vi "LvMPDClient.vi"() -> ()   [LabVIEW 2012]
uses:
  <vilib>/Utility/sysdir.llb/System Directory Type.ctl
  <vilib>/Utility/miscctls.llb/LVPointTypeDef.ctl
  subvi/LvMPDC_Typdef_Setting.ctl
  subvi/LvMPDC_Global_Setting.vi
panel:
  out "Server":string="Title:" caption="Server:"
  out "flag playing":bool
  out "flag connect":bool
  out "flag setting":bool
  out "title":string="LvMPDClient"
  in  "Tree":string(tree)
  in  "List":i32(listbox)
  in  "volume":i32(slide) scale=0.0..100.0
  out "Total":string="59:59"
  out "Current":string="59:59"
  in  "Progress":dbl(slide) scale=0.0..272.0
  out "Artist":string="Artist:"
  out "Title":string="Title:" caption="Title:"
  in  "btn pause":bool
  in  "btn stop":bool
  in  "btn next":bool
  in  "btn prev":bool
  in  "btn play":bool
  # "MusicPlayerDaemon"
  # "http://www.musicpd.org/"
  # "file list"
  # "playlist"
  # "/"
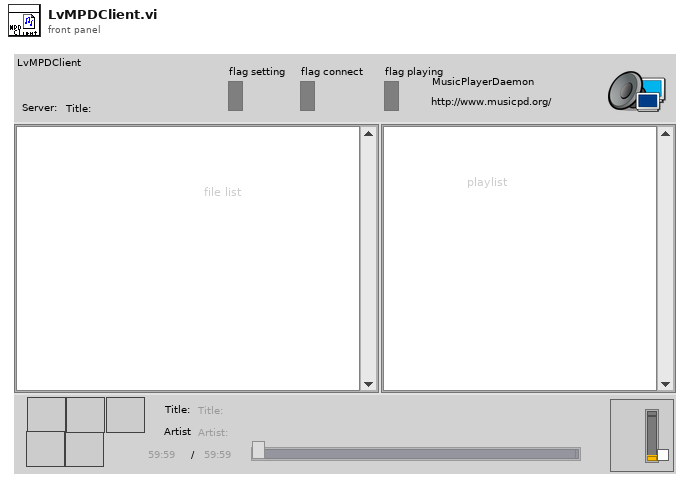
[diagram p1: front panel]
types:
  T1 = typedef "System Directory Type.ctl" = i32
  T2 = typedef "LVPointTypeDef.ctl" = cluster{"Horizontal":i16, "Vertical":i16}
  T3 = cluster{bool, "include Ctrl key?":bool, string}[]
  T4 = typedef "LvMPDC_Typdef_Setting.ctl" = cluster{"Server":string, "Port":u16}
  T5 = cluster{"配列[0]":i16, "配列[1]":i16, "配列[2]":i16, "配列[3]":i16}
  T6 = typedef "LvMPDC_Typdef_status.ctl" = cluster{"volume":i32, "repeat":i32, "random":i32, "single":i32, "consume":i32, "playlist":i32, "playlistlength":i32, "xfade":i32, "mixrampdb":dbl, "mixrampdelay":dbl, "state":enum16{"stop", "play", "pause"}, "song":i32, "songid":i32, "time":dbl, "elapsed":dbl, "bitrate":i32, "audio.samplerate":i32, "audio.bits":i32, "audio.channels":i32, "nextsong":i32, "nextsongid":i32}
  T7 = typedef "LvMPDC_Typdef_currentsong.ctl" = cluster{"file":path, "Last-Modified":string, "time":dbl, "Artist":string, "AlbumArtist":string, "Title":string, "Album":string, "Track":i32, "Date":string, "Genre":string, "Composer":string, "Pos":i32, "Id":i32}
  T8 = typedef "LVRectTypeDef.ctl" = cluster{"Left":i16, "Top":i16, "Right":i16, "Bottom":i16}
  T9 = enum32{"invalid app kind", "Development System", "Run Time System", "Student Edition", "Embedded LabVIEW", "Evaluation", "Custom"}
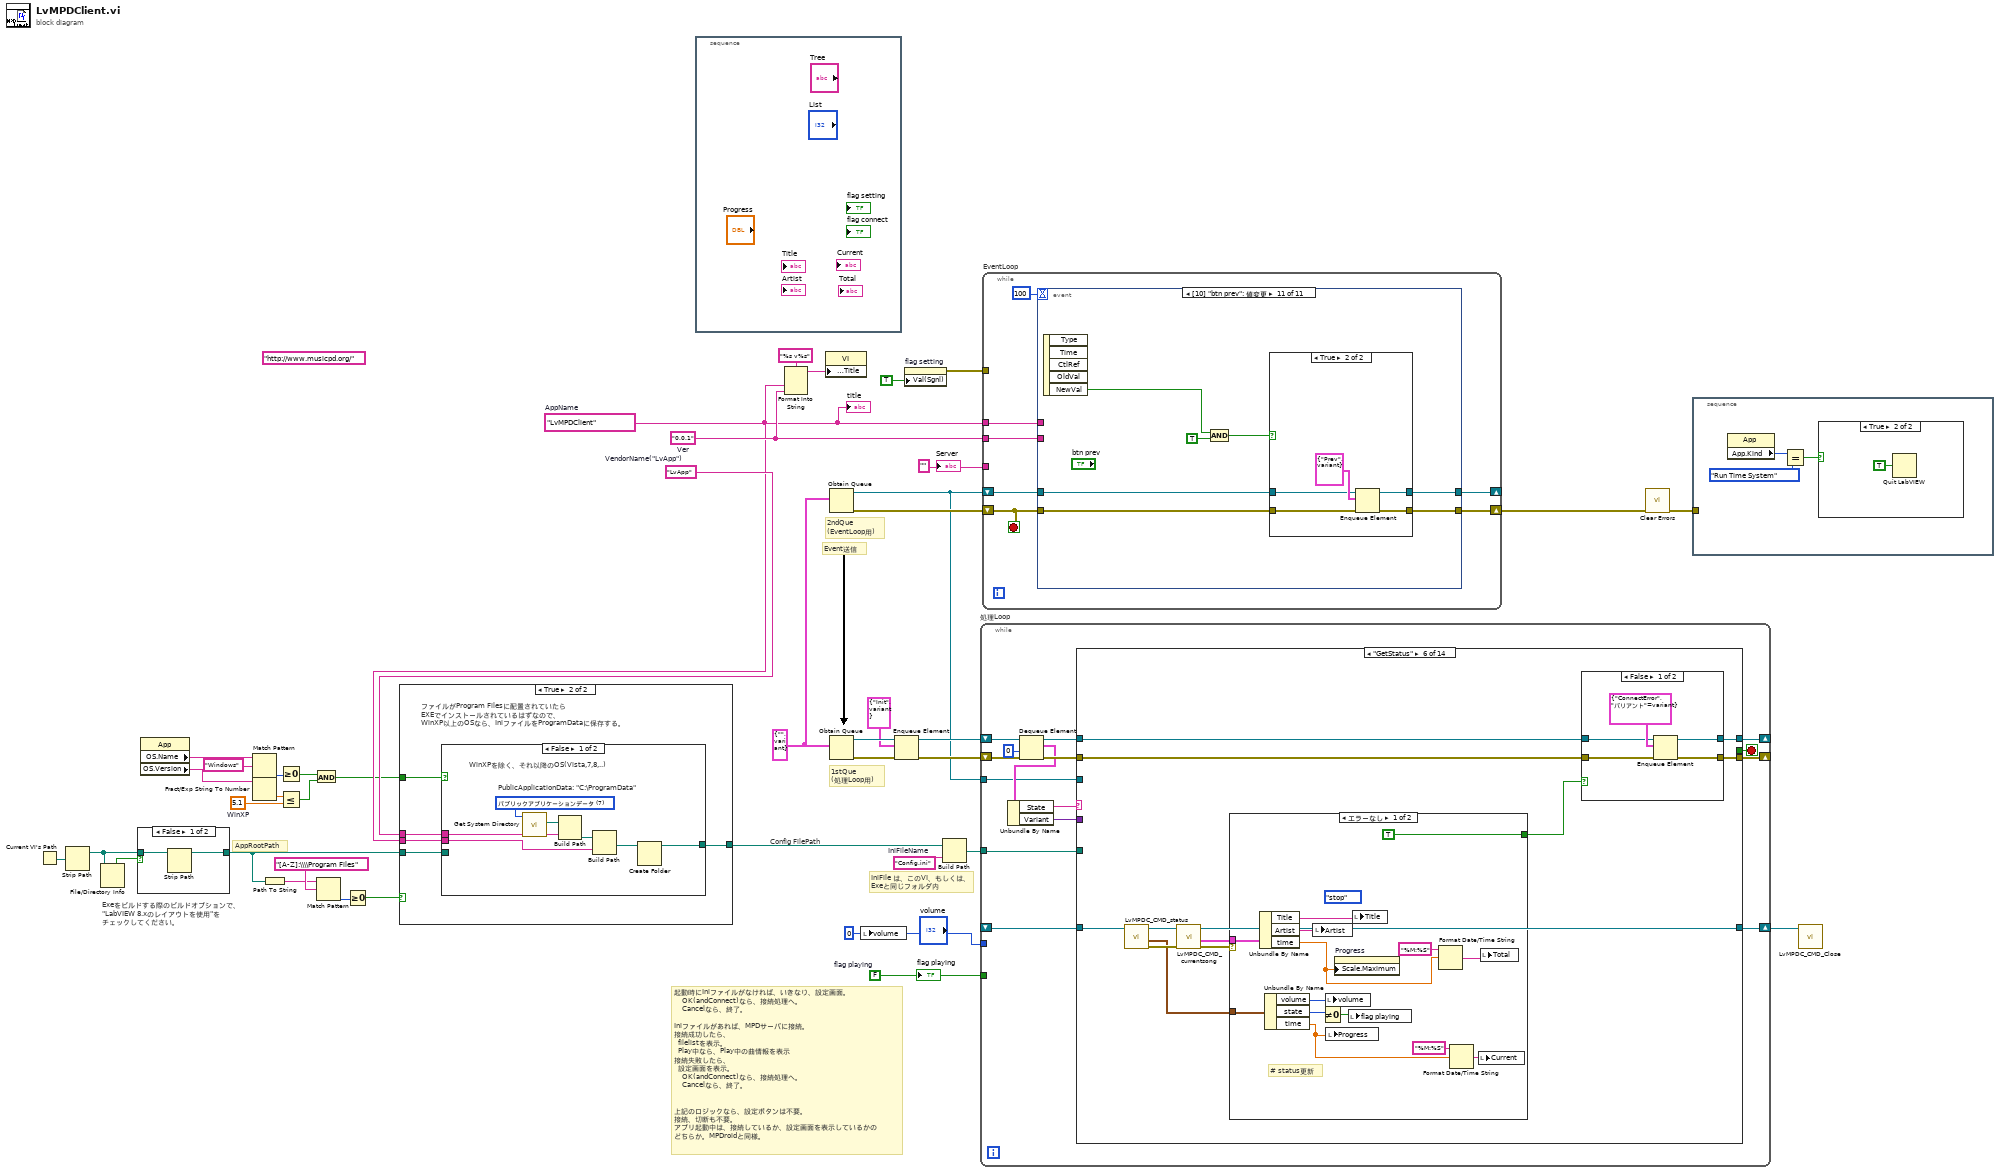
[diagram p0: block diagram]
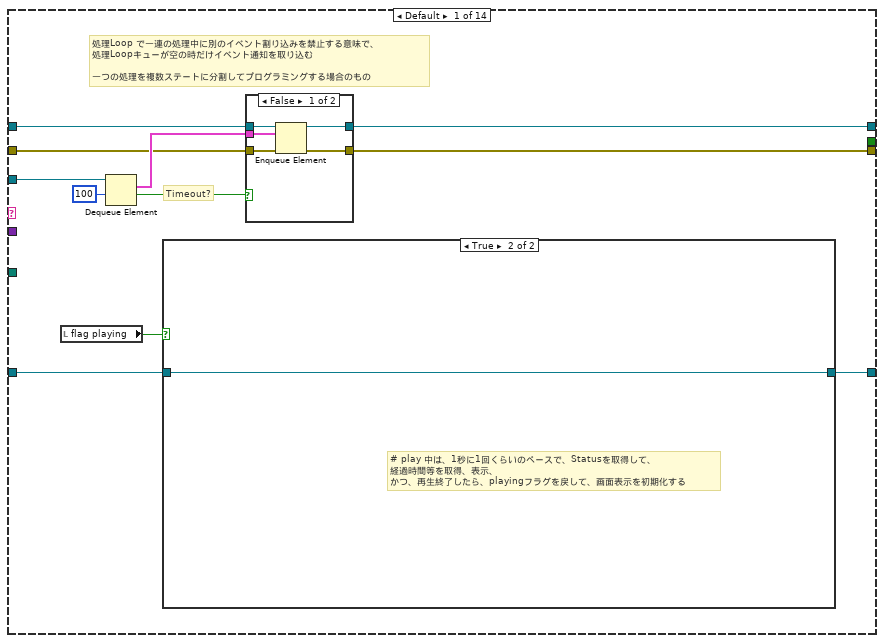
[diagram p6: hidden frame]
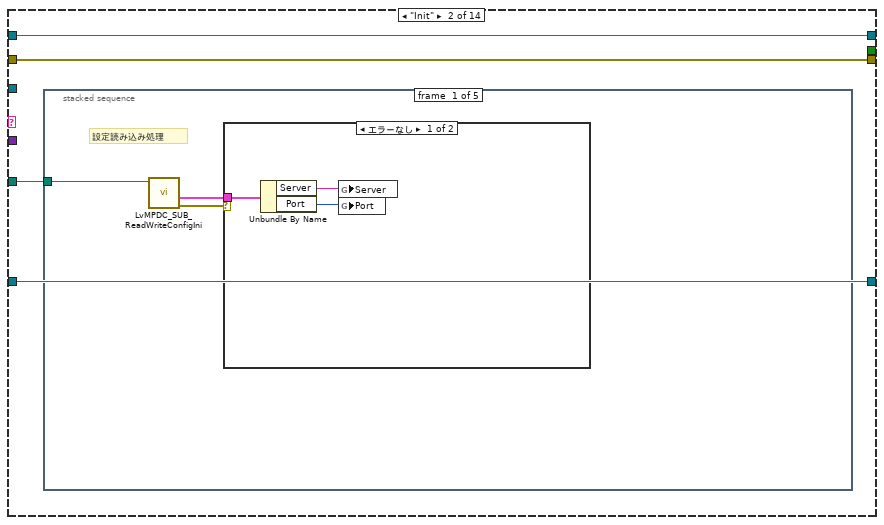
[diagram p9: hidden frame]
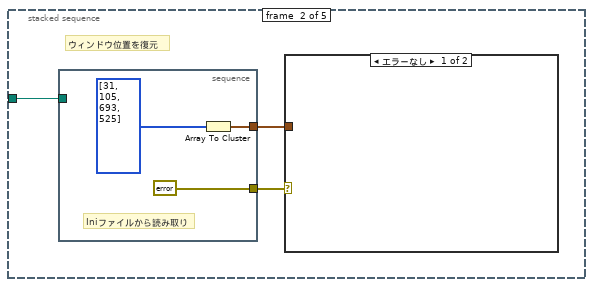
[diagram p11: hidden frame]
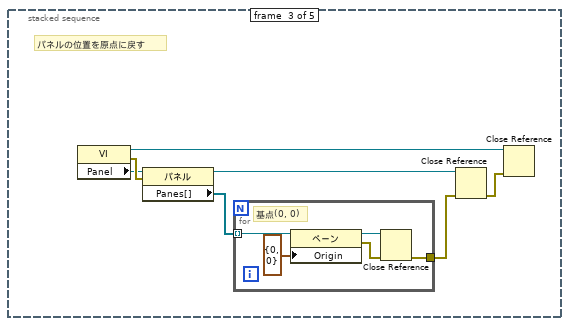
[diagram p13: hidden frame]
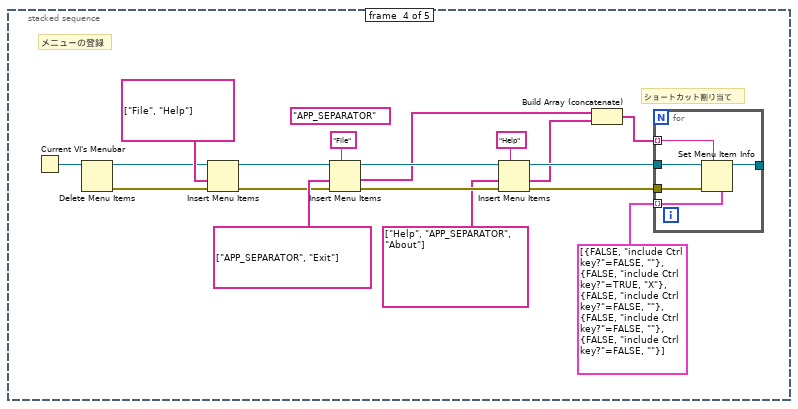
[diagram p14: hidden frame]
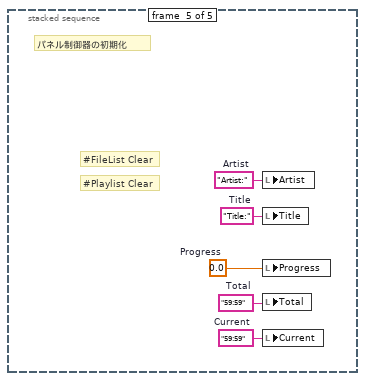
[diagram p15: hidden frame]
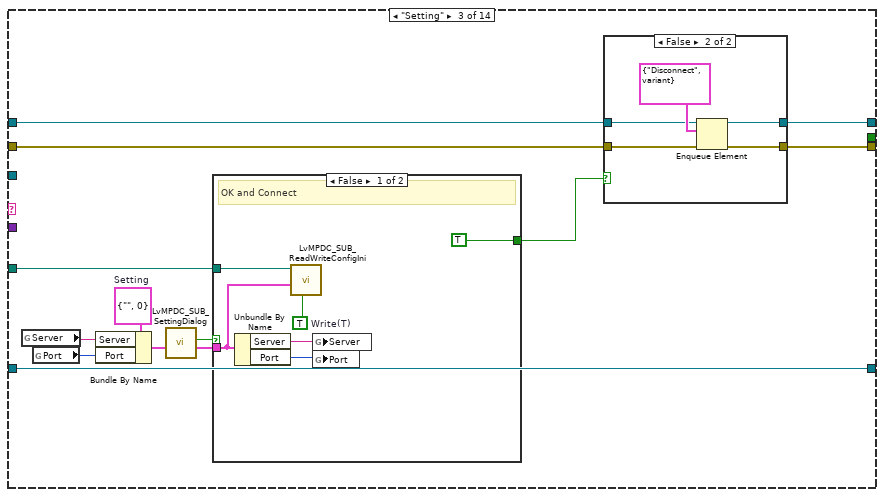
[diagram p16: hidden frame]
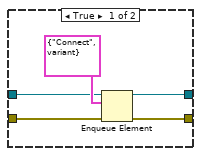
[diagram p17: hidden frame]
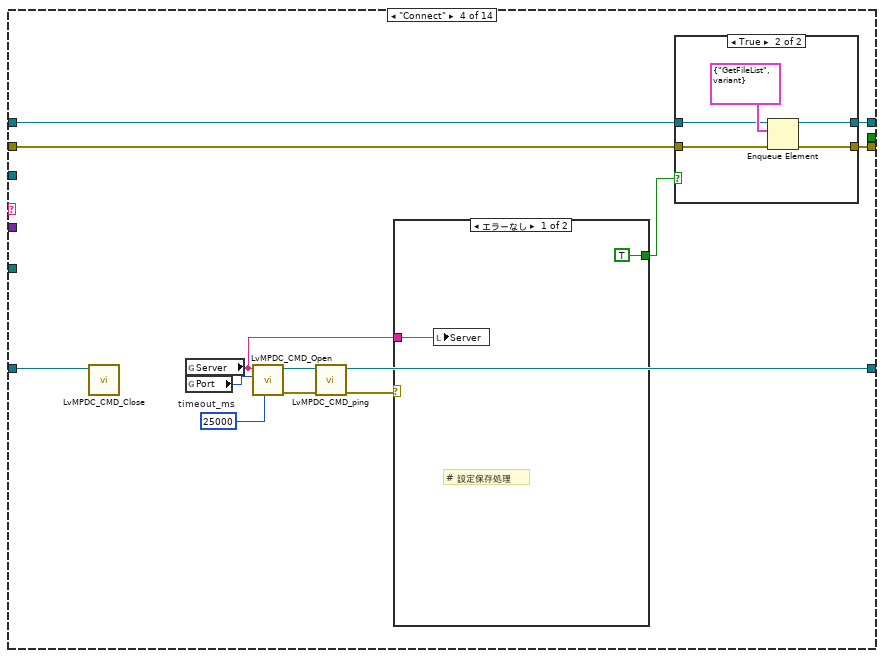
[diagram p19: hidden frame]
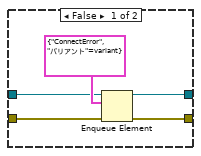
[diagram p20: hidden frame]
diagram:
  w1 = 0 ("volume")
  w2 = "" ("Server")
  w3 = FALSE  # flag playing
  (unwired) "http://www.musicpd.org/" ("aboud MPD")
  w17 = "LvApp"  # VendorName("LvApp")
  w22 = 5.1  # WinXP
  w27 = "Config.ini"  # IniFileName
  w30 = "0.0.1"  # Ver
  w16 = "LvMPDClient"  # AppName
  w41 = cluster{"State":string, "Variant":variant} {"State"="", "Variant"=variant}
  # "起動時にIniファイルがなければ、いきなり、設定画面。\n    OK(andConnect)なら、接続処理へ。\n    Cancelなら、終了。\n\nIniファイルがあれば、MPDサーバに接続。\n接続成功したら、\n  filelistを表示。\n  Play中なら、Play中の曲情報を表示\n接続失敗したら、\n  設定画面を表示。\n    OK(andConnect)なら、接続処理へ。\n    Cancelなら、終了。\n\n\n上記のロジックなら、設定ボタンは不要。\n接続、切断も不要。\nアプリ起動中は、接続しているか、設定画面を表示しているかの\nどちらか。MPDroidと同様。"
  # "Exeをビルドする際のビルドオプションで、\n\"LabVIEW 8.xのレイアウトを使用\"を\nチェックしてください。"
  # "Config FilePath"
  # "AppRootPath"
  # "IniFile は、このVI、もしくは、\nExeと同じフォルダ内"
  # "2ndQue\n(EventLoop用)"
  # "1stQue\n(処理Loop用)"
  # "Event送信"
  n1 = Current VI's Path() -> (path=w13:path)
  n2 = Strip Path(path=w13) -> (stripped path=w14:path)  [unwired: 1 out]
  n3 = File/Directory Info(path=w14) -> (directory=w15:bool)  [unwired: 1 in, 6 out]
  n4 = case shown="FALSE" w15 {
    tunnel: w14 -> [w43 w44]
    tunnel: [w42 w44] -> w10
    frame False {
      n5 = Strip Path(path=w43) -> (stripped path=w42:path)  [unwired: 1 out]
    }
    frame True {
    }
  }
  n6 = property class="App"() -> ("OS.Name"=w26:string, "OS.Version"=w24:string)  [unwired: 2 in, 2 out]
  n7 = Match Pattern(string=w26, regular expression="Windows" ("正規表現")) -> (offset past match=w21:i32)  [unwired: 1 in, 3 out]
  n8 = Fract/Exp String To Number(string=w24) -> (number=w23:dbl)  [unwired: 3 in, 1 out]
  n9 = Path To String(path=w10) -> (string=w9:string)
  n10 = Greater Or Equal To 0?(x=w21) -> (x >= 0?=w20:bool)
  n11 = Less Or Equal?(x=w23, y=w22) -> (x <= y?=w19:bool)
  n12 = And(x=w20, y=w19) -> (x .and. y?=w12:bool)
  n13 = Match Pattern(string=w9, regular expression="[A-Z]:\\\\Program Files" ("正規表現")) -> (offset past match=w8:i32)  [unwired: 1 in, 3 out]
  n14 = Greater Or Equal To 0?(x=w8) -> (x >= 0?=w7:bool)
  n15 = case shown="TRUE" w7 {
    tunnel: w16 -> [_ w50]
    tunnel: [w45 w48] -> w18
    tunnel: w17 -> [_ w49]
    tunnel: w12 -> [_ w47]
    tunnel: w10 -> [w45 w46]
    frame False {
      # "ファイルがProgram Filesに配置されていなかったら\n開発システムでソースから実行しているか、\nExeで適当なフォルダから実行されているので、\nIniファイルは、EXE, またはTop VI と同じ場所に保存"
    }
    frame True {
      # "ファイルがProgram Filesに配置されていたら\nEXEでインストールされているはずなので、\nWinXP以上のOSなら、IniファイルをProgramDataに保存する。"
      n16 = case shown="FALSE" w47 {
        tunnel: w50 -> [w54 _]
        tunnel: w49 -> [w52 _]
        tunnel: [w51 w58] -> w48
        tunnel: w46 -> [_ w58]
        frame False {
          w57 = T1 7 items=["ユーザホーム"=0, "ユーザデスクトップ"=1, "ユーザドキュメント"=2, "ユーザアプリケーションデータ"=3, "ユーザ設定"=4, "ユーザ一時"=5, "パブリックドキュメント"=6, "パブリックアプリケーションデータ"=7, "パブリック環境設定"=8, "パブリックキャッシュ"=13, "システムコアライブラリ"=9, "システムインストールされたライブラリ"=10, "アプリケーションファイル"=11, "ブート容量ルート"=12] ("system directory type")
          # "PublicApplicationData: \"C:\\ProgramData\""
          # "WinXPを除く、それ以降のOS(Vista,7,8,..)"
          n17 = call <vilib>:"Get System Directory.vi"("system directory type"=w57) -> ("system directory"=w56:path)  [unwired: 10 in]
          n18 = Build Path(base path=w56, name or relative path=w52) -> (appended path=w55:path)
          n19 = Build Path(base path=w55, name or relative path=w54) -> (appended path=w53:path)
          n20 = Create Folder(path (use dialog)=w53) -> (created path=w51:path)  [unwired: 2 in, 2 out]
        }
        frame True {
        }
      }
    }
  }
  n21 = stacked-sequence {
    frame #0 {
    }
  }
  n22 = Format Into String(format string="%s v%s" ("形式文字列"), w16, w30) -> (resulting string=w28:string)  [unwired: 2 in, 1 out]
  n23 = property class="VI"("Front Panel.Title"=w28) -> ()  [unwired: 2 in, 2 out]
  n24 = Obtain Queue(element data type=w41) -> (queue out=w34:refnum<queue>, error out=w40:errorcluster)  [unwired: 4 in, 1 out]
  n25 = Obtain Queue(element data type=w41) -> (queue out=w39:refnum<queue>, error out=w37:errorcluster)  [unwired: 4 in, 1 out]
  n26 = local write "volume"(w1) -> ()
  n27 = Enqueue Element(queue=w39, element=cluster{string, "バリアント":variant} {"Init", "バリアント"=variant}, error in (no error)=w37) -> (queue out=w38:refnum<queue>, error out=w36:errorcluster)  [unwired: 1 in, 1 out]
  n28 = property on="flag setting" class="Bool （指定）"("Val(Sgnl)"=TRUE) -> (error out=w5:errorcluster)  [unwired: 2 in, 1 out]
  n29 = Build Path(base path=w18, name or relative path=w27) -> (appended path=w31:path)
  n30 = while "処理Loop" {
    shift-right: [w68] -> _
    shift-left: w38 -> [w73]
    shift-right: [w67] -> _
    shift-left: w36 -> [w70]
    tunnel: w34 -> [w63]
    tunnel: w31 -> [w61]
    shift-right: [w60] -> w4
    shift-left: _ -> [w59]
    tunnel: w3 -> [_]
    tunnel: w1 -> [_]
    stop <- w62 stop-if-true
    n31 = Dequeue Element(queue=w73, timeout in ms (-1)=0 ("タイムアウト（ms）（-1）"), error in (no error)=w70) -> (queue out=w72:refnum<queue>, element=w66:cluster{"State":string, "Variant":variant}, error out=w69:errorcluster)  [unwired: 1 out]
    n32 = Unbundle By Name(w66) -> ("State"=w65:string, "Variant"=w64:variant)
    n33 = case shown="\"GetStatus\"" w65 {
      tunnel: w72 -> [w81 w97 w159 w186 w208 w233 w271 w297 w323 w348 w373 w396 w401 w411]
      tunnel: w63 -> [w84 _ _ _ _ _ _ _ _ _ _ _ _ w409]
      tunnel: w69 -> [w79 w96 w157 w185 w207 w232 w270 w296 w322 w347 w372 w395 w400 w408]
      tunnel: [w80 w97 w158 w184 w206 w231 w269 w295 w321 w346 w371 w393 w398 refnum<queue> refnum ("queue out")] -> w68
      tunnel: [w78 w96 w156 w183 w205 w230 w268 w294 w320 w345 w370 w394 w399 w407] -> w67
      tunnel: w64 -> [_ _ _ _ _ _ _ _ _ _ _ _ _ _]
      tunnel: [_ _ _ _ _ _ _ _ _ _ _ _ _ TRUE] -> w62
      tunnel: w61 -> [_ w95 w150 _ _ _ _ _ _ _ _ _ _ w406]
      tunnel: [w75 w94 w160 w189 w209 w225 w265 w291 w317 w342 w367 w392 w403 w405] -> w60
      tunnel: w59 -> [w76 w94 w160 w188 w209 w228 w266 w292 w318 w343 w368 w392 w404 w405]
      frame Default {
        # "Timeout?"
        # "処理Loop で一連の処理中に別のイベント割り込みを禁止する意味で、\n処理Loopキューが空の時だけイベント通知を取り込む\n\n一つの処理を複数ステートに分割してプログラミングする場合のもの"
        n34 = local read "flag playing"() -> (w74:bool)
        n35 = Dequeue Element(queue=w84, timeout in ms (-1)=100 ("タイムアウト（ms）（-1）")) -> (element=w82:cluster{"State":string, "Variant":variant}, timed out?=w77:bool)  [unwired: 1 in, 2 out]
        n36 = case shown="TRUE" w74 {
          tunnel: w76 -> [w85 w86]
          tunnel: [w85 w86] -> w75
          frame False {
          }
          frame True {
            # "# play 中は、1秒に1回くらいのペースで、Statusを取得して、\n経過時間等を取得、表示、\nかつ、再生終了したら、playingフラグを戻して、画面表示を初期化する"
          }
        }
        n37 = case shown="FALSE" w77 {
          tunnel: w82 -> [w91 _]
          tunnel: w81 -> [w90 w93]
          tunnel: [w89 w93] -> w80
          tunnel: w79 -> [w88 w92]
          tunnel: [w87 w92] -> w78
          frame False {
            n38 = Enqueue Element(queue=w90, element=w91, error in (no error)=w88) -> (queue out=w89:refnum<queue>, error out=w87:errorcluster)  [unwired: 1 in, 1 out]
          }
          frame True {
          }
        }
      }
      frame "Init" {
        n39 = stacked-sequence {
          tunnel: w95 -> [w100 w104 _ _ _]
          frame #0 {
            # "設定読み込み処理"
            n40 = call "LvMPDC_SUB_ReadWriteConfigIni.vi"("ConfigIni filepath"=w100) -> ("error out"=w99:errorcluster, "Config out"=w98:T4)  [unwired: 9 in]
            n41 = case shown="エラーなし" w99 {
              tunnel: w98 -> [w101 _]
              frame No Error {
                n42 = Unbundle By Name(w101) -> ("Server"=w103:string, "Port"=w102:u16)
                n43 = global write "LvMPDC_Global_Setting.vi" "Server"(w103) -> ()
                n44 = global write "LvMPDC_Global_Setting.vi" "Port"(w102) -> ()
              }
              frame Error {
              }
            }
          }
          frame #1 {
            # "ウィンドウ位置を復元"
            n45 = stacked-sequence {
              tunnel: [w107] -> w106
              tunnel: [errorcluster {"status"=FALSE, "code"=0, "source"=""} ("error in (no error)")] -> w105
              tunnel: w104 -> [_]
              frame #0 {
                # "Iniファイルから読み取り"
                n46 = Array To Cluster(array=i16[] [31, 105, 693, 525] ("配列")) -> (cluster=w107:T5)
              }
            }
            n47 = case shown="エラーなし" w105 {
              tunnel: w106 -> [_ _]
              frame No Error {
              }
              frame Error {
              }
            }
          }
          frame #2 {
            # "パネルの位置を原点に戻す"
            n48 = property class="VI"() -> (reference out=w113:refnum<vi>, error out=w116:errorcluster, "Panel"=w110:refnum<vi>)  [unwired: 2 in]
            n49 = property on="プロパティノード" class="パネル"(reference=w110, error in=w116) -> (reference out=w112:refnum<vi>, "Panes[]"=w111:refnum<vi>[])  [unwired: 1 out]
            n50 = for {
              tunnel: w111 -> [w121] mode=indexing
              tunnel: [w118] -> w114
              # "基点(0, 0)"
              n51 = property on="プロパティノード" class="ペーン"(reference=w121, "Origin"=T2 {"Horizontal"=0, "Vertical"=0} ("原点")) -> (reference out=w120:refnum<vi>, error out=w119:errorcluster)  [unwired: 1 in]
              n52 = Close Reference(reference=w120, error in (no error)=w119) -> (error out=w118:errorcluster)
            }
            n53 = Close Reference(reference=w112, error in (no error)=w114) -> (error out=w115:errorcluster)
            n54 = Close Reference(reference=w113, error in (no error)=w115) -> ()  [unwired: 1 out]
          }
          frame #3 {
            (unwired) "APP_SEPARATOR"
            # "ショートカット割り当て"
            # "メニューの登録"
            n55 = Current VI's Menubar() -> (w130:refnum<k9>)
            n56 = Delete Menu Items(9:w130) -> (0:w132:errorcluster, 3:w131:refnum<k9>)  [unwired: 3 in]
            n57 = Insert Menu Items(6:w132, 7:string[] ["File", "Help"] ("item tags"), 9:w131) -> (0:w136:errorcluster, 3:w135:refnum<k9>)  [unwired: 3 in, 1 out]
            n58 = Insert Menu Items(5:"File" ("menu tag"), 6:w136, 7:string[] ["APP_SEPARATOR", "Exit"] ("item tags"), 9:w135) -> (0:w139:errorcluster, 1:w125:string[], 3:w138:refnum<k9>)  [unwired: 2 in]
            n59 = Insert Menu Items(5:"Help" ("menu tag"), 6:w139, 7:string[] ["Help", "APP_SEPARATOR", "About"] ("item tags"), 9:w138) -> (0:w126:errorcluster, 1:w124:string[], 3:w127:refnum<k9>)  [unwired: 2 in]
            n60 = Build Array (concatenate)(w125, w124) -> (w122:string[])
            n61 = for {
              tunnel: w127 -> [w144]
              tunnel: w126 -> [w143]
              tunnel: [w142] -> _
              tunnel: T3 [{FALSE, "include Ctrl key?"=FALSE, ""}, {FALSE, "include Ctrl key?"=TRUE, "X"}, {FALSE, "include Ctrl key?"=FALSE, ""}, {FALSE, "include Ctrl key?"=FALSE, ""}, {FALSE, "include Ctrl key?"=FALSE, ""}] -> [w141] mode=indexing
              tunnel: w122 -> [w140] mode=indexing
              n62 = Set Menu Item Info(4:w141, 7:w140, 8:w143, 11:w144) -> (3:w142:refnum<k9>)  [unwired: 3 in, 1 out]
            }
          }
          frame #4 {
            w145 = "59:59"  # Current
            w146 = "59:59"  # Total
            w147 = 0.0  # Progress
            w148 = "Title:"  # Title
            w149 = "Artist:"  # Artist
            # "#Playlist Clear"
            # "#FileList Clear"
            # "パネル制御器の初期化"
            n63 = local write "Artist"(w149) -> ()
            n64 = local write "Title"(w148) -> ()
            n65 = local write "Progress"(w147) -> ()
            n66 = local write "Total"(w146) -> ()
            n67 = local write "Current"(w145) -> ()
          }
        }
      }
      frame "Setting" {
        w153 = T4 {"Server"="", "Port"=0}  # Setting
        n68 = global read "LvMPDC_Global_Setting.vi" "Server"() -> (w152:string)
        n69 = global read "LvMPDC_Global_Setting.vi" "Port"() -> (w151:u16)
        n70 = Bundle By Name(cluster=w153, "Server"=w152, "Port"=w151) -> (w154:T4)
        n71 = call "LvMPDC_SUB_SettingDialog.vi"("Setting"=w154) -> ("Setting out"=w162:T4, "Caccel?"=w161:bool)  [unwired: 9 in]
        n72 = case shown="FALSE" w161 {
          tunnel: w162 -> [w175 _]
          tunnel: [TRUE _] -> w155
          tunnel: w150 -> [w174 _]
          frame False {
            w173 = TRUE  # Write(T)
            # "OK and Connect"
            n73 = Unbundle By Name(w175) -> ("Server"=w177:string, "Port"=w176:u16)
            n74 = call "LvMPDC_SUB_ReadWriteConfigIni.vi"("Read/Write(T)"=w173, "Config"=w175, "ConfigIni filepath"=w174) -> ()  [unwired: 7 in, 2 out]
            n75 = global write "LvMPDC_Global_Setting.vi" "Server"(w177) -> ()
            n76 = global write "LvMPDC_Global_Setting.vi" "Port"(w176) -> ()
          }
          frame True {
            # "Cancel"
          }
        }
        n77 = case shown="FALSE" w155 {
          tunnel: w159 -> [w166 w171]
          tunnel: [w165 w170] -> w158
          tunnel: w157 -> [w164 w169]
          tunnel: [w163 w168] -> w156
          frame True {
            n78 = Enqueue Element(queue=w166, element=cluster{string, "バリアント":variant} {"Connect", "バリアント"=variant}, error in (no error)=w164) -> (queue out=w165:refnum<queue>, error out=w163:errorcluster)  [unwired: 1 in, 1 out]
          }
          frame False {
            n79 = Enqueue Element(queue=w171, element=cluster{string, "バリアント":variant} {"Disconnect", "バリアント"=variant}, error in (no error)=w169) -> (queue out=w170:refnum<queue>, error out=w168:errorcluster)  [unwired: 1 in, 1 out]
          }
        }
      }
      frame "Connect" {
        w180 = 25000  # timeout_ms
        n80 = call "LvMPDC_CMD_Close.vi"("Connect ID"=w188) -> ()  [unwired: 10 in, 1 out]
        n81 = global read "LvMPDC_Global_Setting.vi" "Server"() -> (w179:string)
        n82 = global read "LvMPDC_Global_Setting.vi" "Port"() -> (w181:u16)
        n83 = call "LvMPDC_CMD_Open.vi"("timeout_ms"=w180, "Port"=w181, "Server"=w179) -> ("error out"=w190:errorcluster, "Connect ID out"=w191:refnum<k5>)  [unwired: 7 in]
        n84 = call "LvMPDC_CMD_ping.vi"("error in (no error)"=w190, "Connect ID"=w191) -> ("error out"=w187:errorcluster, "Connect ID out"=w189:refnum<k5>)  [unwired: 8 in]
        n85 = case shown="エラーなし" w187 {
          tunnel: [TRUE _] -> w182
          tunnel: w179 -> [w202 _]
          frame No Error {
            # "# 設定保存処理"
            n86 = local write "Server"(w202) -> ()
          }
          frame Error {
          }
        }
        n87 = case shown="TRUE" w182 {
          tunnel: w186 -> [w195 w200]
          tunnel: [w194 w199] -> w184
          tunnel: w185 -> [w193 w198]
          tunnel: [w192 w197] -> w183
          frame False {
            n88 = Enqueue Element(queue=w195, element=cluster{string, "バリアント":variant} {"ConnectError", "バリアント"=variant}, error in (no error)=w193) -> (queue out=w194:refnum<queue>, error out=w192:errorcluster)  [unwired: 1 in, 1 out]
          }
          frame True {
            n89 = Enqueue Element(queue=w200, element=cluster{string, "バリアント":variant} {"GetFileList", "バリアント"=variant}, error in (no error)=w198) -> (queue out=w199:refnum<queue>, error out=w197:errorcluster)  [unwired: 1 in, 1 out]
          }
        }
      }
      frame "GetFileList" {
        w210 = errorcluster {"status"=FALSE, "code"=0, "source"=""}  # error IO
        n90 = case shown="エラーなし" w210 {
          tunnel: [TRUE _] -> w204
          frame No Error {
            # "# playlist更新"
          }
          frame Error {
          }
        }
        n91 = case shown="TRUE" w204 {
          tunnel: w208 -> [w214 w219]
          tunnel: [w213 w218] -> w206
          tunnel: w207 -> [w212 w217]
          tunnel: [w211 w216] -> w205
          frame False {
            n92 = Enqueue Element(queue=w214, element=cluster{string, "バリアント":variant} {"ConnectError", "バリアント"=variant}, error in (no error)=w212) -> (queue out=w213:refnum<queue>, error out=w211:errorcluster)  [unwired: 1 in, 1 out]
          }
          frame True {
            n93 = Enqueue Element(queue=w219, element=cluster{string, "バリアント":variant} {"GetStatus", "バリアント"=variant}, error in (no error)=w217) -> (queue out=w218:refnum<queue>, error out=w216:errorcluster)  [unwired: 1 in, 1 out]
          }
        }
      }
      frame "GetStatus" {
        n94 = call "LvMPDC_CMD_status.vi"("Connect ID"=w228) -> ("error out"=w226:errorcluster, "status"=w223:T6, "Connect ID out"=w227:refnum<k5>)  [unwired: 8 in]
        n95 = call "LvMPDC_CMD_currentsong.vi"("error in (no error)"=w226, "Connect ID"=w227) -> ("error out"=w224:errorcluster, "currentsong"=w222:T7, "Connect ID out"=w225:refnum<k5>)  [unwired: 7 in]
        n96 = case shown="エラーなし" w224 {
          tunnel: [TRUE _] -> w229
          tunnel: w223 -> [w259 _]
          tunnel: w222 -> [w258 _]
          frame No Error {
            (unwired) enum16{"stop", "play", "pause"}."stop" ("state")
            # "# status更新"
            n97 = Unbundle By Name(w258) -> ("Title"=w257:string, "Artist"=w256:string, "time"=w250:dbl)
            n98 = Unbundle By Name(w259) -> ("volume"=w262:i32, "state"=w261:enum16{"stop", "play", "pause"}, "time"=w255:dbl)
            n99 = local write "Artist"(w256) -> ()
            n100 = Not Equal To 0?(x=w261) -> (x != 0?=w260:bool)
            n101 = local write "volume"(w262) -> ()
            n102 = local write "Progress"(w255) -> ()
            n103 = property on="Progress" class="Slide （指定）"("Scale.Maximum"=w250) -> ()  [unwired: 2 in, 2 out]
            n104 = local write "flag playing"(w260) -> ()
            n105 = local write "Title"(w257) -> ()
            n106 = Format Date/Time String(time format string (%c)="%M:%S" ("時間形式文字列（%c）"), seconds (now)=w250) -> (date/time string=w252:string)  [unwired: 1 in]
            n107 = Format Date/Time String(time format string (%c)="%M:%S" ("時間形式文字列（%c）"), seconds (now)=w255) -> (date/time string=w251:string)  [unwired: 1 in]
            n108 = local write "Current"(w251) -> ()
            n109 = local write "Total"(w252) -> ()
          }
          frame Error {
          }
        }
        n110 = case shown="FALSE" w229 {
          tunnel: w233 -> [w237 w242]
          tunnel: [w236 w241] -> w231
          tunnel: w232 -> [w235 w240]
          tunnel: [w234 w239] -> w230
          frame False {
            n111 = Enqueue Element(queue=w237, element=cluster{string, "バリアント":variant} {"ConnectError", "バリアント"=variant}, error in (no error)=w235) -> (queue out=w236:refnum<queue>, error out=w234:errorcluster)  [unwired: 1 in, 1 out]
          }
          frame True {
            n112 = disable-structure shown="無効" {
              disable-tunnel: w242 -> [w246 w249]
              disable-tunnel: [w245 w249] -> w241
              disable-tunnel: w240 -> [w244 w248]
              disable-tunnel: [w243 w248] -> w239
              frame Disabled {
                n113 = Enqueue Element(queue=w246, element=cluster{string, "バリアント":variant} {"GetStatus", "バリアント"=variant}, error in (no error)=w244) -> (queue out=w245:refnum<queue>, error out=w243:errorcluster)  [unwired: 1 in, 1 out]
              }
              frame Enabled {
              }
            }
          }
        }
      }
      frame "Play" {
        n114 = call "LvMPDC_CMD_play.vi"("Connect ID"=w266) -> ("error out"=w264:errorcluster, "Connect ID out"=w265:refnum<k5>)  [unwired: 9 in]
        n115 = case shown="エラーなし" w264 {
          tunnel: [TRUE _] -> w267
          frame No Error {
            n116 = local write "flag playing"(TRUE ("flag playing")) -> ()
          }
          frame Error {
          }
        }
        n117 = case shown="FALSE" w267 {
          tunnel: w271 -> [w275 w280]
          tunnel: [w274 w279] -> w269
          tunnel: w270 -> [w273 w278]
          tunnel: [w272 w277] -> w268
          frame False {
            n118 = Enqueue Element(queue=w275, element=cluster{string, "バリアント":variant} {"ConnectError", "バリアント"=variant}, error in (no error)=w273) -> (queue out=w274:refnum<queue>, error out=w272:errorcluster)  [unwired: 1 in, 1 out]
          }
          frame True {
            n119 = disable-structure shown="無効" {
              disable-tunnel: w280 -> [w284 w287]
              disable-tunnel: [w283 w287] -> w279
              disable-tunnel: w278 -> [w282 w286]
              disable-tunnel: [w281 w286] -> w277
              frame Disabled {
                n120 = Enqueue Element(queue=w284, element=cluster{string, "バリアント":variant} {"GetStatus", "バリアント"=variant}, error in (no error)=w282) -> (queue out=w283:refnum<queue>, error out=w281:errorcluster)  [unwired: 1 in, 1 out]
              }
              frame Enabled {
              }
            }
          }
        }
      }
      frame "Stop" {
        n121 = call "LvMPDC_CMD_stop.vi"("Connect ID"=w292) -> ("error out"=w290:errorcluster, "Connect ID out"=w291:refnum<k5>)  [unwired: 9 in]
        n122 = case shown="エラーなし" w290 {
          tunnel: [TRUE _] -> w293
          frame No Error {
            n123 = local write "flag playing"(FALSE ("flag playing")) -> ()
          }
          frame Error {
          }
        }
        n124 = case shown="FALSE" w293 {
          tunnel: w297 -> [w301 w306]
          tunnel: [w300 w305] -> w295
          tunnel: w296 -> [w299 w304]
          tunnel: [w298 w303] -> w294
          frame False {
            n125 = Enqueue Element(queue=w301, element=cluster{string, "バリアント":variant} {"ConnectError", "バリアント"=variant}, error in (no error)=w299) -> (queue out=w300:refnum<queue>, error out=w298:errorcluster)  [unwired: 1 in, 1 out]
          }
          frame True {
            n126 = disable-structure shown="無効" {
              disable-tunnel: w306 -> [w310 w313]
              disable-tunnel: [w309 w313] -> w305
              disable-tunnel: w304 -> [w308 w312]
              disable-tunnel: [w307 w312] -> w303
              frame Disabled {
                n127 = Enqueue Element(queue=w310, element=cluster{string, "バリアント":variant} {"GetStatus", "バリアント"=variant}, error in (no error)=w308) -> (queue out=w309:refnum<queue>, error out=w307:errorcluster)  [unwired: 1 in, 1 out]
              }
              frame Enabled {
              }
            }
          }
        }
      }
      frame "Pause" {
        n128 = call "LvMPDC_CMD_pause.vi"("Connect ID"=w318) -> ("error out"=w316:errorcluster, "Connect ID out"=w317:refnum<k5>)  [unwired: 9 in]
        n129 = case shown="エラーなし" w316 {
          tunnel: [TRUE _] -> w319
          frame No Error {
          }
          frame Error {
          }
        }
        n130 = case shown="FALSE" w319 {
          tunnel: w323 -> [w327 w332]
          tunnel: [w326 w331] -> w321
          tunnel: w322 -> [w325 w330]
          tunnel: [w324 w329] -> w320
          frame False {
            n131 = Enqueue Element(queue=w327, element=cluster{string, "バリアント":variant} {"ConnectError", "バリアント"=variant}, error in (no error)=w325) -> (queue out=w326:refnum<queue>, error out=w324:errorcluster)  [unwired: 1 in, 1 out]
          }
          frame True {
            n132 = disable-structure shown="無効" {
              disable-tunnel: w332 -> [w336 w339]
              disable-tunnel: [w335 w339] -> w331
              disable-tunnel: w330 -> [w334 w338]
              disable-tunnel: [w333 w338] -> w329
              frame Disabled {
                n133 = Enqueue Element(queue=w336, element=cluster{string, "バリアント":variant} {"GetStatus", "バリアント"=variant}, error in (no error)=w334) -> (queue out=w335:refnum<queue>, error out=w333:errorcluster)  [unwired: 1 in, 1 out]
              }
              frame Enabled {
              }
            }
          }
        }
      }
      frame "Next" {
        n134 = call "LvMPDC_CMD_next.vi"("Connect ID"=w343) -> ("error out"=w341:errorcluster, "Connect ID out"=w342:refnum<k5>)  [unwired: 9 in]
        n135 = case shown="エラーなし" w341 {
          tunnel: [TRUE _] -> w344
          frame No Error {
          }
          frame Error {
          }
        }
        n136 = case shown="FALSE" w344 {
          tunnel: w348 -> [w352 w357]
          tunnel: [w351 w356] -> w346
          tunnel: w347 -> [w350 w355]
          tunnel: [w349 w354] -> w345
          frame False {
            n137 = Enqueue Element(queue=w352, element=cluster{string, "バリアント":variant} {"ConnectError", "バリアント"=variant}, error in (no error)=w350) -> (queue out=w351:refnum<queue>, error out=w349:errorcluster)  [unwired: 1 in, 1 out]
          }
          frame True {
            n138 = disable-structure shown="無効" {
              disable-tunnel: w357 -> [w361 w364]
              disable-tunnel: [w360 w364] -> w356
              disable-tunnel: w355 -> [w359 w363]
              disable-tunnel: [w358 w363] -> w354
              frame Disabled {
                n139 = Enqueue Element(queue=w361, element=cluster{string, "バリアント":variant} {"GetStatus", "バリアント"=variant}, error in (no error)=w359) -> (queue out=w360:refnum<queue>, error out=w358:errorcluster)  [unwired: 1 in, 1 out]
              }
              frame Enabled {
              }
            }
          }
        }
      }
      frame "Prev" {
        n140 = call "LvMPDC_CMD_previous.vi"("Connect ID"=w368) -> ("error out"=w366:errorcluster, "Connect ID out"=w367:refnum<k5>)  [unwired: 9 in]
        n141 = case shown="エラーなし" w366 {
          tunnel: [TRUE _] -> w369
          frame No Error {
          }
          frame Error {
          }
        }
        n142 = case shown="FALSE" w369 {
          tunnel: w373 -> [w377 w382]
          tunnel: [w376 w381] -> w371
          tunnel: w372 -> [w375 w380]
          tunnel: [w374 w379] -> w370
          frame False {
            n143 = Enqueue Element(queue=w377, element=cluster{string, "バリアント":variant} {"ConnectError", "バリアント"=variant}, error in (no error)=w375) -> (queue out=w376:refnum<queue>, error out=w374:errorcluster)  [unwired: 1 in, 1 out]
          }
          frame True {
            n144 = disable-structure shown="無効" {
              disable-tunnel: w382 -> [w386 w389]
              disable-tunnel: [w385 w389] -> w381
              disable-tunnel: w380 -> [w384 w388]
              disable-tunnel: [w383 w388] -> w379
              frame Disabled {
                n145 = Enqueue Element(queue=w386, element=cluster{string, "バリアント":variant} {"GetStatus", "バリアント"=variant}, error in (no error)=w384) -> (queue out=w385:refnum<queue>, error out=w383:errorcluster)  [unwired: 1 in, 1 out]
              }
              frame Enabled {
              }
            }
          }
        }
      }
      frame "ConnectError" {
        w391 = "Failure. MPD Server connection"  # メッセージ
        n146 = One Button Dialog(message=w391) -> ()  [unwired: 1 in, 1 out]
        n147 = Enqueue Element(queue=w396, element=cluster{string, "バリアント":variant} {"Setting", "バリアント"=variant}, error in (no error)=w395) -> (queue out=w393:refnum<queue>, error out=w394:errorcluster)  [unwired: 1 in, 1 out]
      }
      frame "Disconnect" {
        w403 = refnum<k5> refnum  # Connect ID out
        n148 = call "LvMPDC_CMD_Close.vi"("Connect ID"=w404) -> ()  [unwired: 10 in, 1 out]
        n149 = Enqueue Element(queue=w401, element=cluster{string, "バリアント":variant} {"Final", "バリアント"=variant}, error in (no error)=w400) -> (queue out=w398:refnum<queue>, error out=w399:errorcluster)  [unwired: 1 in, 1 out]
      }
      frame "Final" {
        n150 = stacked-sequence {
          tunnel: w406 -> [w414]
          frame #0 {
            n151 = property class="VI"() -> ("Front Panel.PanelBounds"=w413:T8)  [unwired: 2 in, 2 out]
            n152 = stacked-sequence {
              tunnel: w414 -> [_]
              tunnel: w413 -> [w415]
              frame #0 {
                # "現在のWindow位置を\nIniファイルに保存"
                n153 = Cluster To Array(cluster=w415) -> ()  [unwired: 1 out]
              }
            }
          }
        }
        n154 = Release Queue(queue=w411, error in (no error)=w408) -> (error out=w407:errorcluster)  [unwired: 1 in, 2 out]
        n155 = Release Queue(queue=w409) -> ()  [unwired: 2 in, 3 out]
      }
    }
  }
  n156 = while "EventLoop" {
    shift-right: [w420] -> _
    shift-left: w34 -> [w421]
    shift-right: [w419] -> w33
    shift-left: w40 -> [w418]
    tunnel: w16 -> [w417]
    tunnel: w30 -> [w416]
    tunnel: w5 -> [_]
    tunnel: w2 -> [_]
    stop <- w418 stop-if-true
    n157 = event shown="[10] \"btn prev\": 値変更" {
      selector: _ -> [_ _ _ _ _ _ _ _ _ _ _]
      dyn-events: _ -> [_ _ _ _ _ _ _ _ _ _ _]
      timeout: 100 -> [_ _ _ _ _ _ _ _ _ _ _]
      tunnel: w421 -> [w426 w432 w438 w446 w465 w478 w493 w507 w521 w535 w549]
      tunnel: [w423 w431 w437 w445 w464 w477 w492 w506 w520 w534 w548] -> w420
      tunnel: w418 -> [w425 w430 w436 w444 w466 w479 w494 w508 w522 w536 w550]
      tunnel: [w424 w429 w435 w443 w463 w476 w491 w505 w519 w533 w547] -> w419
      tunnel: w417 -> [_ _ _ w441 _ _ _ _ _ _ _]
      tunnel: w416 -> [_ _ _ w440 _ _ _ _ _ _ _]
      event Timeout {
        # "EventLoopの終了用"
        # "Que解放をチェック\n(終了?)"
        n158 = event-data() -> ()  [unwired: 1 in, 2 out]
        n159 = Get Queue Status(queue=w426, error in (no error)=w425) -> (queue out=w423:refnum<queue>, error out=w424:errorcluster)  [unwired: 1 in, 6 out]
      }
      event Application Instance Close? {
        n160 = event-data() -> ()  [unwired: 1 in, 4 out]
        n161 = Enqueue Element(queue=w432, element=cluster{string, "バリアント":variant} {"Disconnect", "バリアント"=variant}, error in (no error)=w430) -> (queue out=w431:refnum<queue>, error out=w429:errorcluster)  [unwired: 1 in, 1 out]
        n162 = event-data("SilentShutdown"=TRUE, "Discard?"=FALSE ("破棄?")) -> ()  [unwired: 1 in, 1 out]
      }
      event Panel Close? {
        n163 = event-data() -> ()  [unwired: 1 in, 3 out]
        n164 = Enqueue Element(queue=w438, element=cluster{string, "バリアント":variant} {"Disconnect", "バリアント"=variant}, error in (no error)=w436) -> (queue out=w437:refnum<queue>, error out=w435:errorcluster)  [unwired: 1 in, 1 out]
        n165 = event-data("Discard?"=TRUE) -> ()  [unwired: 1 in, 1 out]
      }
      event Menu Selection (User) {
        n166 = event-data() -> ("ItemPath"=w442:string)  [unwired: 1 in, 5 out]
        n167 = case shown="デフォルト" w442 {
          tunnel: w446 -> [w448 w453 w459 w461]
          tunnel: [w448 w452 w459 w461] -> w445
          tunnel: w444 -> [w447 w451 w458 w460]
          tunnel: [w447 w450 w458 w460] -> w443
          tunnel: w441 -> [_ _ w457 _]
          tunnel: w440 -> [_ _ w456 _]
          frame Default {
          }
          frame "File:Exit" {
            n168 = Enqueue Element(queue=w453, element=cluster{string, "バリアント":variant} {"Final", "バリアント"=variant}, error in (no error)=w451) -> (queue out=w452:refnum<queue>, error out=w450:errorcluster)  [unwired: 1 in, 1 out]
          }
          frame "Help:About" {
            n169 = Format Into String(format string="%s\n\nVersion : %s" ("メッセージ"), w457, w456) -> (resulting string=w454:string)  [unwired: 2 in, 1 out]
            n170 = One Button Dialog(message=w454) -> ()  [unwired: 1 in, 1 out]
          }
          frame "Help:Help" {
          }
        }
      }
      event "flag setting": Value Change {
        n171 = event-data() -> ("NewVal"=w462:bool)  [unwired: 1 in, 4 out]
        n172 = case shown="TRUE" w462 {
          tunnel: w466 -> [w467 w473]
          tunnel: w465 -> [w468 w472]
          tunnel: [w468 w471] -> w464
          tunnel: [w467 w470] -> w463
          frame False {
          }
          frame True {
            n173 = local write "flag setting"(FALSE) -> ()
            n174 = Enqueue Element(queue=w472, element=cluster{string, "バリアント":variant} {"Setting", "バリアント"=variant}, error in (no error)=w473) -> (queue out=w471:refnum<queue>, error out=w470:errorcluster)  [unwired: 1 in, 1 out]
          }
        }
      }
      event "flag connect": Value Change {
        n175 = event-data() -> ("NewVal"=w475:bool)  [unwired: 1 in, 4 out]
        n176 = case shown="TRUE" w475 {
          tunnel: w479 -> [w480 w485]
          tunnel: w478 -> [w481 w484]
          tunnel: [w481 w483] -> w477
          tunnel: [w480 w482] -> w476
          frame False {
          }
          frame True {
            n177 = Enqueue Element(queue=w484, element=cluster{string, "バリアント":variant} {"Connect", "バリアント"=variant}, error in (no error)=w485) -> (queue out=w483:refnum<queue>, error out=w482:errorcluster)  [unwired: 1 in, 1 out]
          }
        }
      }
      event "btn play": Value Change {
        n178 = event-data() -> ("NewVal"=w488:bool)  [unwired: 1 in, 4 out]
        n179 = local read "flag playing"() -> (w490:bool)
        n180 = Not(x=w490) -> (.not. x?=w489:bool)
        n181 = And(x=w488, y=w489) -> (x .and. y?=w487:bool)
        n182 = case shown="TRUE" w487 {
          tunnel: w494 -> [w495 w500]
          tunnel: w493 -> [w496 w499]
          tunnel: [w496 w498] -> w492
          tunnel: [w495 w497] -> w491
          frame False {
          }
          frame True {
            n183 = Enqueue Element(queue=w499, element=cluster{string, "バリアント":variant} {"Play", "バリアント"=variant}, error in (no error)=w500) -> (queue out=w498:refnum<queue>, error out=w497:errorcluster)  [unwired: 1 in, 1 out]
          }
        }
      }
      event "btn stop": Value Change {
        n184 = event-data() -> ("NewVal"=w504:bool)  [unwired: 1 in, 4 out]
        n185 = local read "flag playing"() -> (w502:bool)
        n186 = And(x=w504, y=w502) -> (x .and. y?=w503:bool)
        n187 = case shown="TRUE" w503 {
          tunnel: w508 -> [w509 w514]
          tunnel: w507 -> [w510 w513]
          tunnel: [w510 w512] -> w506
          tunnel: [w509 w511] -> w505
          frame False {
          }
          frame True {
            n188 = Enqueue Element(queue=w513, element=cluster{string, "バリアント":variant} {"Stop", "バリアント"=variant}, error in (no error)=w514) -> (queue out=w512:refnum<queue>, error out=w511:errorcluster)  [unwired: 1 in, 1 out]
          }
        }
      }
      event "btn pause": Value Change {
        n189 = event-data() -> ("NewVal"=w518:bool)  [unwired: 1 in, 4 out]
        n190 = local read "flag playing"() -> (w516:bool)
        n191 = And(x=w518, y=w516) -> (x .and. y?=w517:bool)
        n192 = case shown="TRUE" w517 {
          tunnel: w522 -> [w523 w528]
          tunnel: w521 -> [w524 w527]
          tunnel: [w524 w526] -> w520
          tunnel: [w523 w525] -> w519
          frame False {
          }
          frame True {
            n193 = Enqueue Element(queue=w527, element=cluster{string, "バリアント":variant} {"Pause", "バリアント"=variant}, error in (no error)=w528) -> (queue out=w526:refnum<queue>, error out=w525:errorcluster)  [unwired: 1 in, 1 out]
          }
        }
      }
      event "btn next": Value Change {
        n194 = event-data() -> ("NewVal"=w532:bool)  [unwired: 1 in, 4 out]
        n195 = And(x=w532, y=TRUE) -> (x .and. y?=w531:bool)
        n196 = case shown="TRUE" w531 {
          tunnel: w536 -> [w537 w542]
          tunnel: w535 -> [w538 w541]
          tunnel: [w538 w540] -> w534
          tunnel: [w537 w539] -> w533
          frame False {
          }
          frame True {
            n197 = Enqueue Element(queue=w541, element=cluster{string, "バリアント":variant} {"Next", "バリアント"=variant}, error in (no error)=w542) -> (queue out=w540:refnum<queue>, error out=w539:errorcluster)  [unwired: 1 in, 1 out]
          }
        }
      }
      event "btn prev": Value Change {
        n198 = event-data() -> ("NewVal"=w546:bool)  [unwired: 1 in, 4 out]
        n199 = And(x=w546, y=TRUE) -> (x .and. y?=w545:bool)
        n200 = case shown="TRUE" w545 {
          tunnel: w550 -> [w551 w556]
          tunnel: w549 -> [w552 w555]
          tunnel: [w552 w554] -> w548
          tunnel: [w551 w553] -> w547
          frame False {
          }
          frame True {
            n201 = Enqueue Element(queue=w555, element=cluster{string, "バリアント":variant} {"Prev", "バリアント"=variant}, error in (no error)=w556) -> (queue out=w554:refnum<queue>, error out=w553:errorcluster)  [unwired: 1 in, 1 out]
          }
        }
      }
    }
  }
  n202 = call <vilib>:"Clear Errors.vi"("error in (no error)"=w33) -> ("error out"=w32:errorcluster)  [unwired: 6 in]
  n203 = stacked-sequence {
    tunnel: w32 -> [_]
    frame #0 {
      n204 = property class="App"() -> ("App.Kind"=w560:T9)  [unwired: 2 in, 2 out]
      n205 = Equal?(x=w560, y=T9."Run Time System" ("アプリケーション:種類")) -> (x = y?=w558:bool)
      n206 = case shown="TRUE" w558 {
        frame False {
        }
        frame True {
          n207 = Quit LabVIEW(quit? (T)=TRUE ("終了?（T）")) -> ()
        }
      }
    }
  }
  n208 = call "LvMPDC_CMD_Close.vi"("Connect ID"=w4) -> ()  [unwired: 10 in, 1 out]
  "title" <- w16
  "flag playing" <- w3
  "Server" <- w2
